vi "Validate Channel GUIDs.vi"(6 "input GUID":string, 7 "output GUID":string, 8 "error in (no error)":errorcluster, 10 "imported bitfile scalars in":T2[](array[typedef]), 11 "FPGA addon refnum in":T1 format="%.0x") -> (0 "error out":errorcluster, 2 "valid GUIDs?":bool, 3 "FPGA addon refnum out":T1=18446744073709551615 format="%.0x")   [LabVIEW 2021, in "FPGA Addon Bitfile Reload Unit Tests.lvclass"]
uses:
  FPGA Addon Bitfile Reload Unit Tests.lvclass
  <vilib>/NI VeriStand/Custom Device API/Custom Device Item Ref.ctl
  APIs/Scripting API/TypeDefs/Output Scalar Data.ctl
  Addon/Addon Shared/Types/FPGA Addon Data Type.ctl
  <vilib>/NI VeriStand/Custom Device Tools/Custom Device Utility Library/NI VeriStand - Search for Item by Name.vi
  <vilib>/NI VeriStand/Custom Device Tools/Custom Device Utility Library/Custom Device Utility Library.lvlib
  <vilib>/NI VeriStand/Custom Device API/Custom Device API.lvlib
  APIs/Scripting API/Scripting API.lvlib
  Addon/Addon Shared/FPGA Addon Shared.lvlib
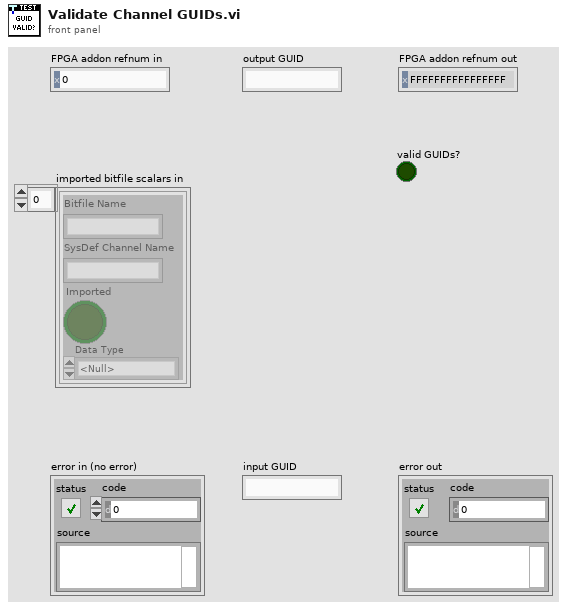
[diagram p1: front panel]
types:
  T1 = typedef "Custom Device API.lvlib/Custom Device Item Ref.ctl" = u64
  T2 = typedef "Scripting API.lvlib/Output Scalar Data.ctl" = cluster{"Bitfile Name":string, "SysDef Channel Name":string, "Imported":bool, "Data Type":T3}
  T3 = typedef "FPGA Addon Shared.lvlib/FPGA Addon Data Type.ctl" = enum8{"<Null>", "I8", "I16", "I32", "I64", "U8", "U16", "U32", "U64", "SGL", "Boolean", "Analog PWM In Settings", "Analog PWM In", "Digital PWM In Settings", "Digital PWM In", "Digital PWM Out", "Sine Out", "FXP", "FXP+/-24.5", "FXP+/-16.5", "FXP+/-32.8", "FXP+/-64.32", "FXP+/-16.7", "FXP+/-20.5", "FXP+/-27.5", "FXP+/-32.16", "FXP+16.3", "FXP+18.3", "Digital Static In", "Digital Static Out", "Digital Static In Settings", "Digital WSS Out", "Quad Encoder Settings", "Quad Encoder In", "Group"}
  T4 = typedef "Custom Device API.lvlib/Custom Device Item Info.ctl" = cluster{"Name":string, "Is Channel":bool, "GUID":string, "Is Waveform":bool}
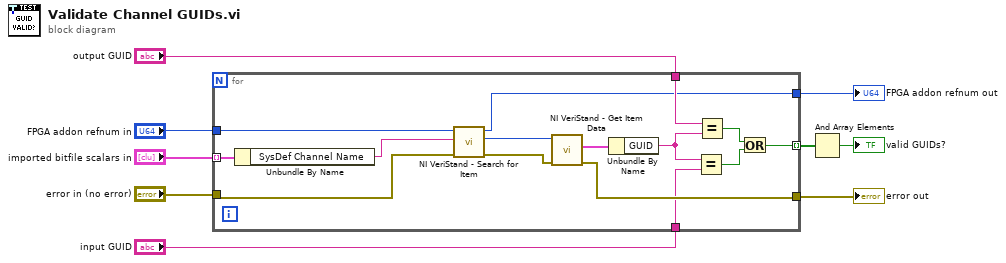
[diagram p0: block diagram]
diagram:
  n1 = for {
    tunnel: "imported bitfile scalars in" -> [w24] mode=indexing
    tunnel: "FPGA addon refnum in" -> [w22]
    tunnel: "error in (no error)" -> [w21]
    tunnel: [w14] -> w2 mode=indexing
    tunnel: [w13] -> w7
    tunnel: "output GUID" -> [w12]
    tunnel: "input GUID" -> [w11]
    tunnel: [w10] -> w3
    n2 = Unbundle By Name(w24) -> ("SysDef Channel Name"=w23:string)
    n3 = call-poly <vilib>:"NI VeriStand - Search for Item.vi"("error in"=w21, "Item Name"=w23, "Section Ref in"=w22) -> ("error out"=w20:errorcluster, "Item Ref"=w19:T1, "Section Ref out"=w10:T1)  [unwired: 5 in, 1 out]
    n4 = call <vilib>:"NI VeriStand - Get Item Data.vi"("error in (no error)"=w20, "Item Ref in"=w19) -> ("error out"=w13:errorcluster, "Item Info"=w18:T4)  [unwired: 6 in, 2 out]
    n5 = Unbundle By Name(w18) -> ("GUID"=w17:string)
    n6 = Equal?(x=w17, y=w11) -> (x = y?=w15:bool)
    n7 = Equal?(x=w12, y=w17) -> (x = y?=w16:bool)
    n8 = Or(x=w16, y=w15) -> (x .or. y?=w14:bool)
  }
  "error out" <- w7
  "FPGA addon refnum out" <- w3
  n9 = And Array Elements(Boolean array=w2) -> (logical AND=→"valid GUIDs?":bool)
